vi "ChangeSession.vi"(1 "error in (no error)":errorcluster, 2 "Session":string="This is line 2{ENTER}This is line ") -> (0 "error out":errorcluster)   [LabVIEW 2014]
panel:
  in  "AutoItX3Lib.IAutoItX3":refnum<k7>
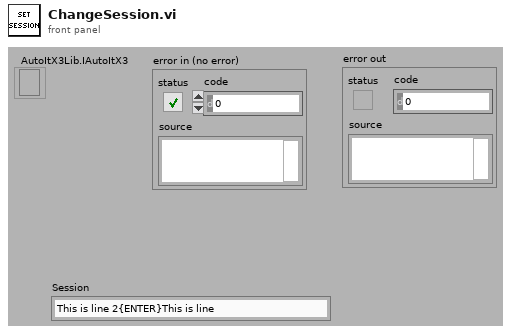
[diagram p1: front panel]
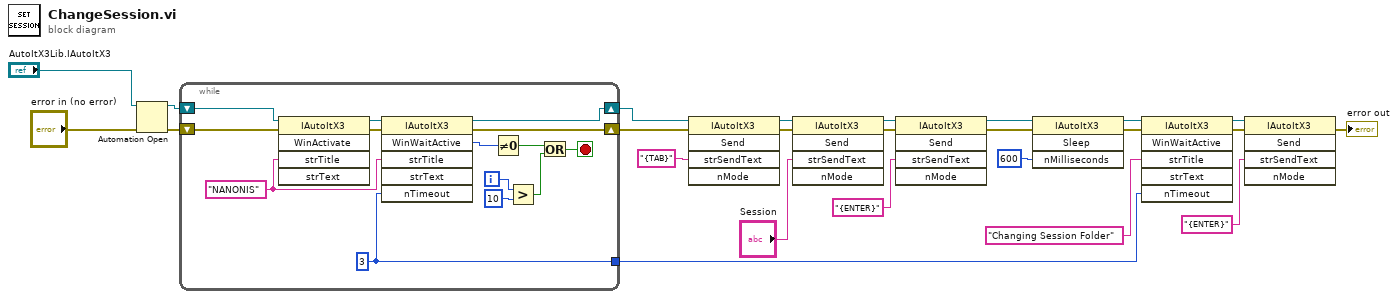
[diagram p0: block diagram]
diagram:
  n1 = Automation Open(error in (no error)="error in (no error)", Automation Refnum="AutoItX3Lib.IAutoItX3") -> (Automation Refnum=w12:refnum<k7>, error out=w13:errorcluster)  [unwired: 2 in]
  n2 = while {
    tunnel: [w31] -> w1
    shift-right: [w37] -> w22
    shift-left: w13 -> [w35]
    shift-right: [w38] -> w23
    shift-left: w12 -> [w33]
    i -> [w29]
    stop <- w25 stop-if-true
    w31 = 3 ("nTimeout")
    w36 = "NANONIS" ("strTitle")
    n3 = invoke class="IAutoItX3" method="WinActivate"(reference=w33, error in=w35, "strTitle"=w36) -> (reference out=w32:refnum<k7>, error out=w34:errorcluster)  [unwired: 2 in, 3 out]
    n4 = invoke class="IAutoItX3" method="WinWaitActive"(reference=w32, error in=w34, "strTitle"=w36, "nTimeout"=w31) -> (reference out=w38:refnum<k7>, error out=w37:errorcluster, "WinWaitActive"=w30:i32)  [unwired: 2 in, 3 out]
    n5 = Not Equal To 0?(x=w30) -> (x != 0?=w27:bool)
    n6 = Greater?(x=w29, y=10) -> (0:w26:bool)
    n7 = Or(x=w27, y=w26) -> (x .or. y?=w25:bool)
  }
  n8 = invoke class="IAutoItX3" method="Send"(reference=w23, error in=w22, "strSendText"="{TAB}" ("strTitle")) -> (reference out=w20:refnum<k7>, error out=w19:errorcluster)  [unwired: 2 in, 3 out]
  n9 = invoke class="IAutoItX3" method="Send"(reference=w20, error in=w19, "strSendText"="Session") -> (reference out=w9:refnum<k7>, error out=w7:errorcluster)  [unwired: 2 in, 3 out]
  n10 = invoke class="IAutoItX3" method="Send"(reference=w9, error in=w7, "strSendText"="{ENTER}") -> (reference out=w8:refnum<k7>, error out=w6:errorcluster)  [unwired: 2 in, 3 out]
  n11 = invoke class="IAutoItX3" method="Sleep"(reference=w8, error in=w6, "nMilliseconds"=600) -> (reference out=w5:refnum<k7>, error out=w4:errorcluster)  [unwired: 1 in, 2 out]
  n12 = invoke class="IAutoItX3" method="WinWaitActive"(reference=w5, error in=w4, "strTitle"="Changing Session Folder", "nTimeout"=w1) -> (reference out=w16:refnum<k7>, error out=w15:errorcluster)  [unwired: 2 in, 4 out]
  n13 = invoke class="IAutoItX3" method="Send"(reference=w16, error in=w15, "strSendText"="{ENTER}" ("strTitle")) -> (error out=→"error out":errorcluster)  [unwired: 2 in, 4 out]
